vi "Create From Variant (String).vi"(8 "error in (no error)":errorcluster, 10 "Variant":variant, 11 "JSON String in":refnum<class "JSON Value.lvclass">) -> (0 "error out":errorcluster, 3 "JSON String out":refnum<class "JSON Value.lvclass">)   [LabVIEW 2016, in "JSON Value.lvclass"]
doc: "Creates a new JSON instance from the given Variant."
uses:
  JSON Value.lvclass
  JSON Value.lvclass/JSON Value.ctl
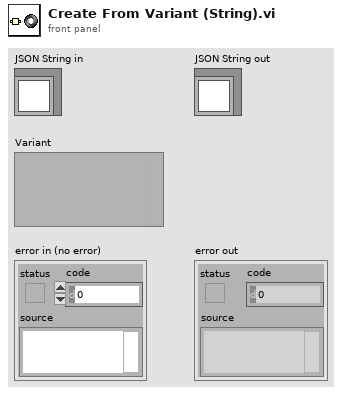
[diagram p1: front panel]
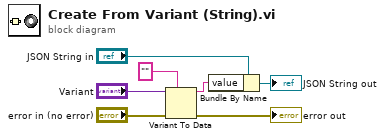
[diagram p0: block diagram]
diagram:
  n1 = Variant To Data(error in="error in (no error)", type="", Variant="Variant") -> (data=w3:string, error out=→"error out":errorcluster)
  n2 = Bundle By Name(cluster="JSON String in", "value"=w3) -> (→"JSON String out":refnum<class "JSON Value.lvclass">)
